vi "pp2_updateSideState.vi"(8 "error in (no error)":errorcluster, 9 "refnum in":refnum<file>, 10 "Daq config In":T1={"Sound AO"="Dev2/ao0", "Shock intesity AO"="Dev1/ao1", "Code_LED DO"="Dev1/port1:2", "Switch DI"="Dev1/port0/line0:1", "Webcam"="cam0", "Sound AO task"="", "Sound card task"=0, "Shock intensity AO task"="", "Code_LED DO task"="", "Switch DI task"="", "AO <=> Sound card"=FALSE, "Sound card"=0, "sample rate"=8000.0, "Variable shock"=FALSE, "Webcam on"=FALSE, "Tone gate PFI"="/Dev1/PFI1", "Waveform memo"={"t0"=timestamp(0 s since 1904-01-01), "dt"=1.0, "Y"=[]}} {"sample rate" min=8000.0; "Sound card task" format="%.0x"}, 11 "State In":T4={"Curr  tr"=0, "Curr (ms)"=0, "Cum (ms)"=0, "Run loop diff"=0, "Tone countdown (ms)"=0, "Countdown (ms)"=0, "Curr State"=enum."0 NULL", "Prev State"=enum."1 Habituation", "Null"=FALSE, "Sw"=FALSE, "Tone\nGate"=FALSE, "Stim"=FALSE, "Current DAQ DO Int"=0, "Current Loaded Trial"={"Trial Type Number"=1, "Trial Type"=enum."GO", "Trial Weight"=100, "Shock (mA)"=0.3, "Duration (ms)"=0.25, "Sound Type"=enum."04 FM Sweep", "Stim P1"=4000.0, "Stim P2"=0.0, "Stim P3"=0.0, "Stim P4"=2000.0}, "Next Trial (for display purposes)"={"Trial Type Number"=1, "Trial Type"=enum."GO", "Trial Weight"=100, "Shock (mA)"=0.3, "Duration (ms)"=0.25, "Sound Type"=enum."04 FM Sweep", "Stim P1"=4000.0, "Stim P2"=0.0, "Stim P3"=0.0, "Stim P4"=2000.0}, "Total trials memo"=0, "State start cum memo (ms)"=0, "Last dur jump time memo (ms)"=0, "Last dur shock time memo (ms)"=0, "Tone repeat memo"=0, "Webcam on"=FALSE, "Webcam recording"=FALSE} {"Current DAQ DO Int" format="%b"; "Next Trial (for display purposes)"."Shock (mA)" min=-1.0 max=5.0; "Next Trial (for display purposes)"."Trial Weight" step=1; "Next Trial (for display purposes)"."Duration (ms)" min=0.0 max=1.0; "Next Trial (for display purposes)"."Trial Type Number" min=1 step=1; "Current Loaded Trial"."Shock (mA)" min=-1.0 max=5.0; "Current Loaded Trial"."Trial Weight" step=1; "Current Loaded Trial"."Duration (ms)" min=0.0 max=1.0; "Current Loaded Trial"."Trial Type Number" min=1 step=1}) -> (0 "error out":errorcluster, 2 "Daq config Out":T1={"Sound AO"="Dev2/ao0", "Shock intesity AO"="Dev1/ao1", "Code_LED DO"="Dev1/port1:2", "Switch DI"="Dev1/port0/line0:1", "Webcam"="cam0", "Sound AO task"="", "Sound card task"=0, "Shock intensity AO task"="", "Code_LED DO task"="", "Switch DI task"="", "AO <=> Sound card"=FALSE, "Sound card"=0, "sample rate"=8000.0, "Variable shock"=FALSE, "Webcam on"=FALSE, "Tone gate PFI"="/Dev1/PFI1", "Waveform memo"={"t0"=timestamp(0 s since 1904-01-01), "dt"=1.0, "Y"=[]}} {"sample rate" min=8000.0; "Sound card task" format="%.0x"}, 3 "State Out":T4={"Curr  tr"=0, "Curr (ms)"=0, "Cum (ms)"=0, "Run loop diff"=0, "Tone countdown (ms)"=0, "Countdown (ms)"=0, "Curr State"=enum."0 NULL", "Prev State"=enum."1 Habituation", "Null"=FALSE, "Sw"=FALSE, "Tone\nGate"=FALSE, "Stim"=FALSE, "Current DAQ DO Int"=0, "Current Loaded Trial"={"Trial Type Number"=1, "Trial Type"=enum."GO", "Trial Weight"=100, "Shock (mA)"=0.3, "Duration (ms)"=0.25, "Sound Type"=enum."04 FM Sweep", "Stim P1"=4000.0, "Stim P2"=0.0, "Stim P3"=0.0, "Stim P4"=2000.0}, "Next Trial (for display purposes)"={"Trial Type Number"=1, "Trial Type"=enum."GO", "Trial Weight"=100, "Shock (mA)"=0.3, "Duration (ms)"=0.25, "Sound Type"=enum."04 FM Sweep", "Stim P1"=4000.0, "Stim P2"=0.0, "Stim P3"=0.0, "Stim P4"=2000.0}, "Total trials memo"=0, "State start cum memo (ms)"=0, "Last dur jump time memo (ms)"=0, "Last dur shock time memo (ms)"=0, "Tone repeat memo"=0, "Webcam on"=FALSE, "Webcam recording"=FALSE} {"Current DAQ DO Int" format="%b"; "Next Trial (for display purposes)"."Shock (mA)" min=-1.0 max=5.0; "Next Trial (for display purposes)"."Trial Weight" step=1; "Next Trial (for display purposes)"."Duration (ms)" min=0.0 max=1.0; "Next Trial (for display purposes)"."Trial Type Number" min=1 step=1; "Current Loaded Trial"."Shock (mA)" min=-1.0 max=5.0; "Current Loaded Trial"."Trial Weight" step=1; "Current Loaded Trial"."Duration (ms)" min=0.0 max=1.0; "Current Loaded Trial"."Trial Type Number" min=1 step=1}, 4 "State timeout":bool, 6 "Side change":bool)   [LabVIEW 2013]
uses:
  pp2_CTL_StateInfo.ctl
  pp2_CTL_State.ctl
  pp2_Trial.ctl
  pp2_CTL_TrialType.ctl
  labolabo2/waveforms/WFTypes.ctl
  pp2_CTL_DaqConfig.ctl
  <vilib>/userdefined/High Color/IMAQdx.ctl
  <vilib>/sound2/lvsound2.llb/Sound Output Task ID.ctl
  <vilib>/DAQmx/read.llb/DAQmx Read (Digital Bool 1Line 1Point).vi
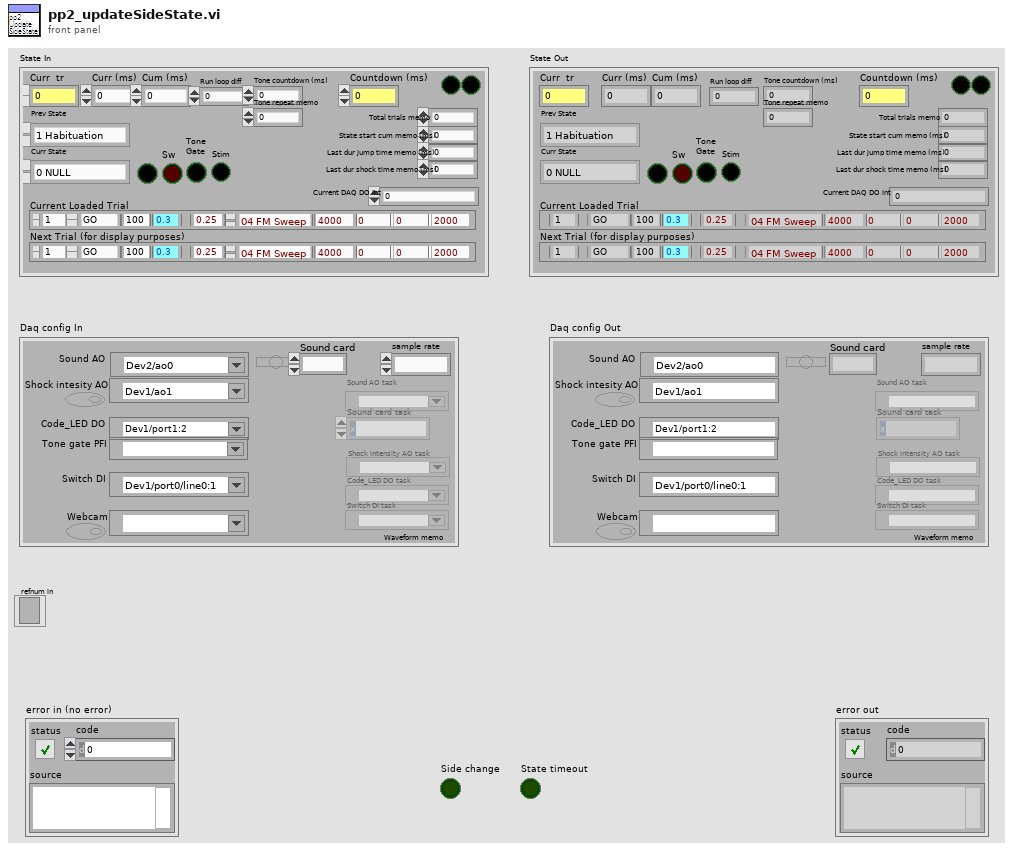
[diagram p1: front panel]
types:
  T1 = typedef "pp2_CTL_DaqConfig.ctl" = cluster{"Sound AO":tag, "Shock intesity AO":tag, "Code_LED DO":tag, "Switch DI":tag, "Webcam":T2, "Sound AO task":refnum<k21>, "Sound card task":T3, "Shock intensity AO task":refnum<k21>, "Code_LED DO task":refnum<k21>, "Switch DI task":refnum<k21>, "AO <=> Sound card":bool, "Sound card":u32, "sample rate":dbl, "Variable shock":bool, "Webcam on":bool, "Tone gate PFI":tag, "Waveform memo":waveform(dbl)}
  T2 = typedef "IMAQdx.ctl" = refnum<k21>
  T3 = typedef "Sound Output Task ID.ctl" = u32
  T4 = typedef "pp2_CTL_StateInfo.ctl" = cluster{"Curr  tr":u16, "Curr (ms)":i64, "Cum (ms)":i64, "Run loop diff":i64, "Tone countdown (ms)":i64, "Countdown (ms)":i64, "Curr State":T5, "Prev State":T5, "Null":bool, "Sw":bool, "Tone\nGate":bool, "Stim":bool, "Current DAQ DO Int":u16, "Current Loaded Trial":T6, "Next Trial (for display purposes)":T6, "Total trials memo":i64, "State start cum memo (ms)":i64, "Last dur jump time memo (ms)":i64, "Last dur shock time memo (ms)":i64, "Tone repeat memo":i64, "Webcam on":bool, "Webcam recording":bool}
  T5 = typedef "pp2_CTL_State.ctl" = enum8{"0 NULL", "1 Habituation", "2 (Load Trial)", "3 Stay Period", "4 Load Audio/Click Delay", "5 GO Trial", "6 GO Jumped", "7 GO Timeout", "8 NOGO Trial", "9 NOGO Jumped", "10 NOGO Timeout", "11 TEST Trial", "12 TEST Jumped", "13 TEST Timeout", "14 Intertrial Interval", "15 Done"}
  T6 = typedef "pp2_Trial.ctl" = cluster{"Trial Type Number":u8, "Trial Type":T7, "Trial Weight":u32, "Shock (mA)":dbl, "Duration (ms)":dbl, "Sound Type":T8, "Stim P1":dbl, "Stim P2":dbl, "Stim P3":dbl, "Stim P4":dbl}
  T7 = typedef "pp2_CTL_TrialType.ctl" = enum16{"OFF", "GO", "NOGO", "TEST"}
  T8 = typedef "WFTypes.ctl" = enum16{"00 NULL", "01 DC", "02 Noise", "03 Pure Tone", "04 FM Sweep"}
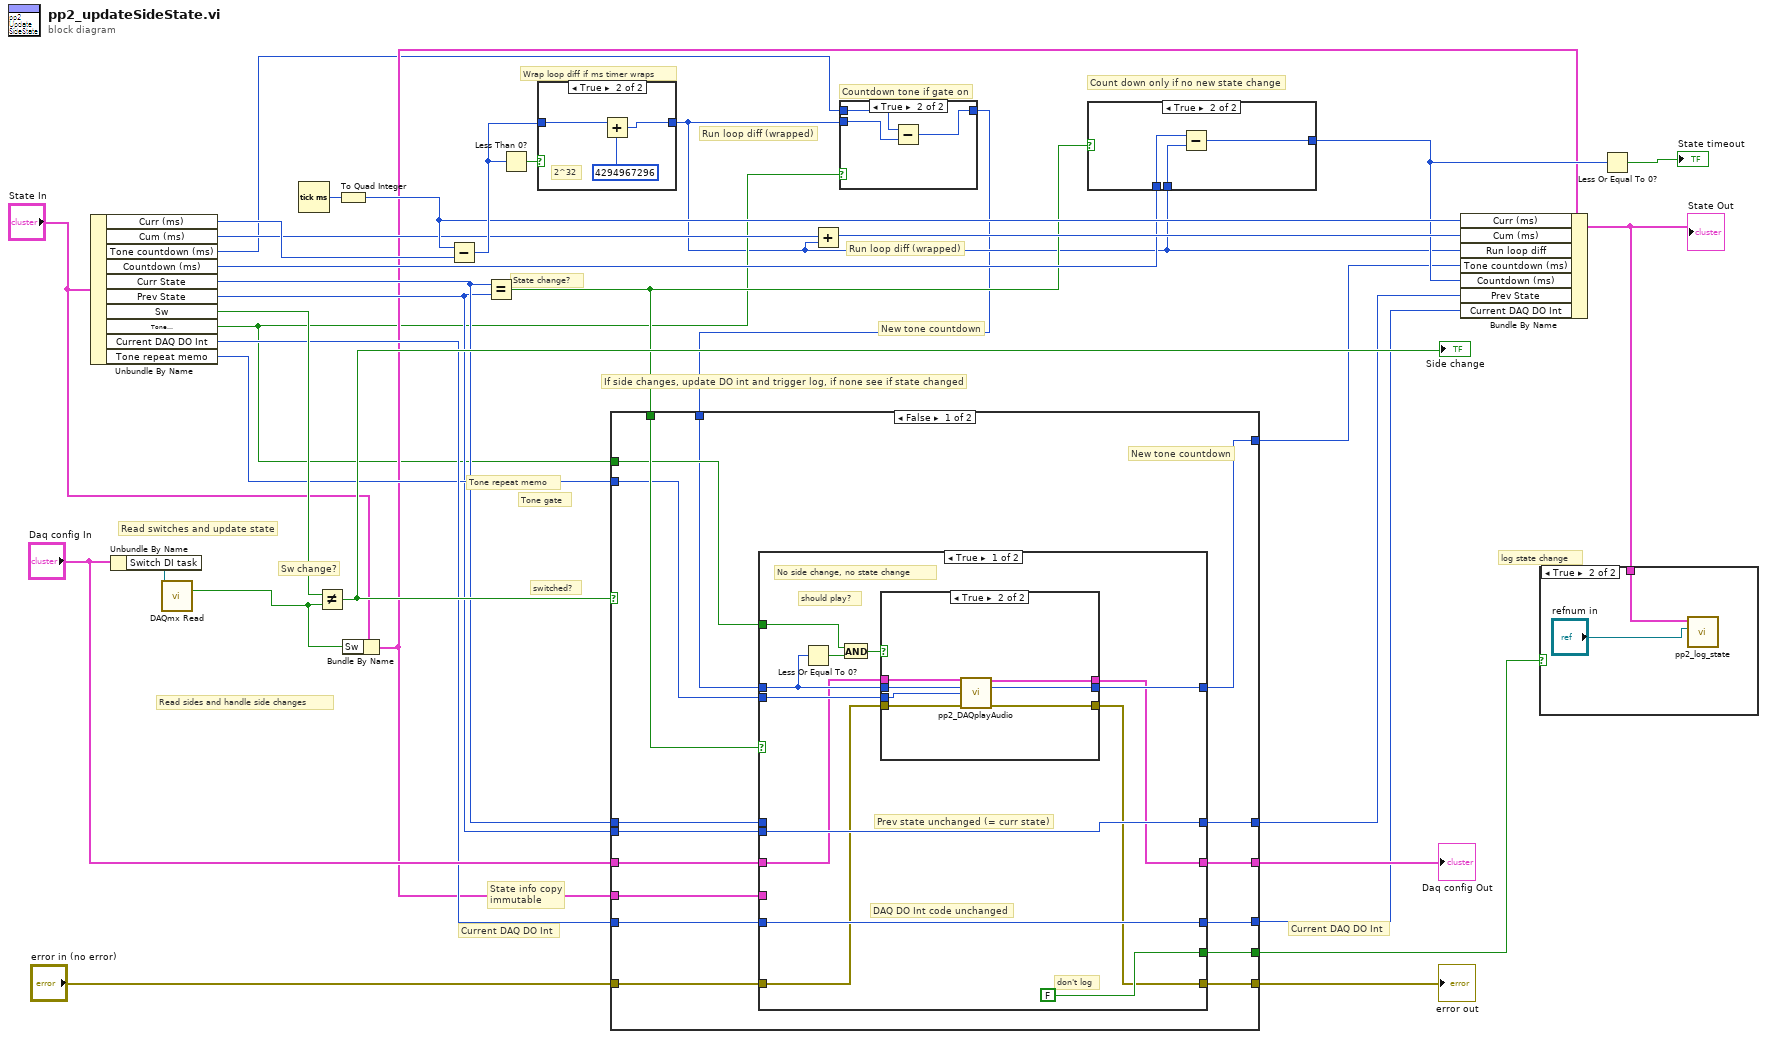
[diagram p0: block diagram]
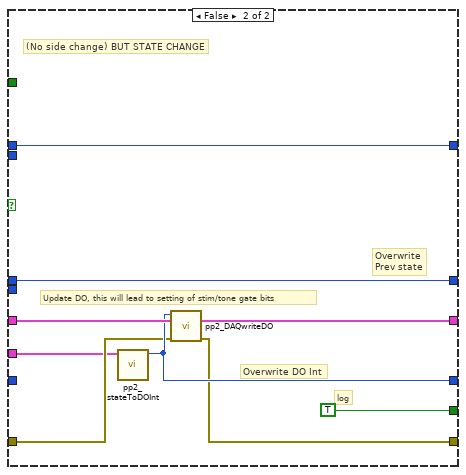
[diagram p6: hidden frame]
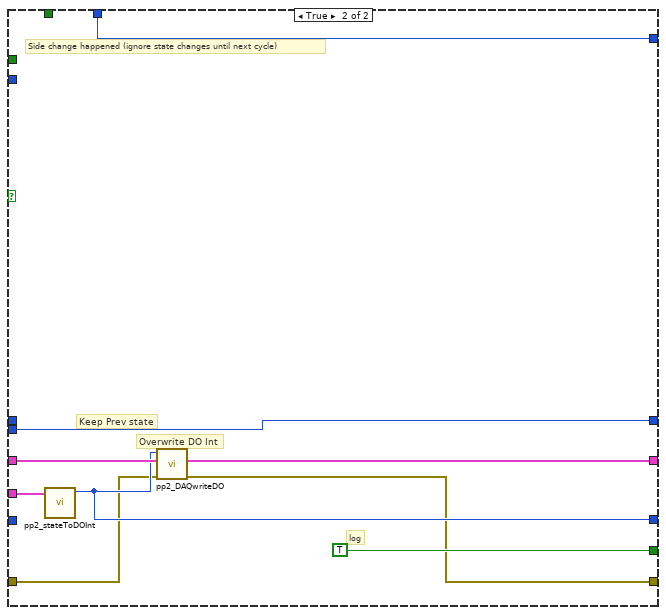
[diagram p7: hidden frame]
diagram:
  # "New tone countdown"
  # "Countdown tone if gate on"
  # "switched?"
  # "Read switches and update state"
  # "State info copy\nimmutable"
  # "Tone repeat memo"
  # "Sw change?"
  # "Run loop diff (wrapped)"
  # "State change?"
  # "Current DAQ DO Int"
  # "Current DAQ DO Int"
  # "Count down only if no new state change"
  # "Tone gate"
  # "Run loop diff (wrapped)"
  # "Wrap loop diff if ms timer wraps"
  # "If side changes, update DO int and trigger log, if none see if state changed"
  # "Read sides and handle side changes"
  # "log state change"
  n1 = Unbundle By Name("State In") -> ("Curr (ms)"=w30:i64, "Cum (ms)"=w29:i64, "Tone countdown (ms)"=w3:i64, "Countdown (ms)"=w27:i64, "Curr State"=w12:T5, "Prev State"=w11:T5, "Sw"=w25:bool, "Tone\nGate"=w5:bool, "Current DAQ DO Int"=w18:u16, "Tone repeat memo"=w13:i64)
  n2 = Unbundle By Name("Daq config In") -> ("Switch DI task"=w26:refnum<k21>)
  n3 = call-poly <vilib>:"DAQmx Read.vi"("task/channels in"=w26) -> ("data"=w1:bool)  [unwired: 12 in, 2 out]
  n4 = Tick Count (ms)() -> (millisecond timer value=w34:u32)
  n5 = Not Equal?(x=w25, y=w1) -> (x != y?=w22:bool)
  "Side change" <- w22
  n6 = To Quad Integer(1:w34) -> (0:w31:i64)
  n7 = Bundle By Name(cluster="State In", "Sw"=w1) -> (w6:T4)
  n8 = Subtract(x=w31, y=w30) -> (x-y=w32:i64)
  n9 = Equal?(x=w12, y=w11) -> (x = y?=w10:bool)
  n10 = Less Than 0?(x=w32) -> (x < 0?=w33:bool)
  n11 = case shown="True" w33 {
    tunnel: w32 -> [w35 w37]
    tunnel: [w35 w38] -> w4
    frame False {
    }
    frame True {
      # "2^32"
      n12 = Add(x=w37, y=i64 4294967296) -> (x+y=w38:i64)
    }
  }
  n13 = Add(x=w29, y=w4) -> (x+y=w28:i64)
  n14 = case shown="True" w5 {
    tunnel: [w39 w40] -> w2
    tunnel: w3 -> [w39 w42]
    tunnel: w4 -> [_ w41]
    frame False {
      # "Passthrough if\ntone gate off"
    }
    frame True {
      n15 = Subtract(x=w42, y=w41) -> (x-y=w40:i64)
    }
  }
  n16 = case shown="False" w22 {
    tunnel: w12 -> [w58 _]
    tunnel: w11 -> [w56 w99]
    tunnel: [w57 w99] -> w21
    tunnel: "Daq config In" -> [w48 w97]
    tunnel: [w54 w95] -> w7
    tunnel: [w53 w96] -> w19
    tunnel: w18 -> [w55 _]
    tunnel: "error in (no error)" -> [w47 w94]
    tunnel: [w51 w93] -> w16
    tunnel: [w52 TRUE] -> w15
    tunnel: w5 -> [w44 _]
    tunnel: w13 -> [w46 _]
    tunnel: w10 -> [w50 _]
    tunnel: w6 -> [w49 w92]
    tunnel: [w45 w91] -> w9
    tunnel: w2 -> [w43 w91]
    frame False {
      # "New tone countdown"
      n17 = case shown="True" w50 {
        tunnel: w58 -> [_ w90]
        tunnel: [w71 w90] -> w57
        tunnel: w56 -> [w71 _]
        tunnel: w55 -> [w70 _]
        tunnel: [w70 w87] -> w54
        tunnel: w48 -> [w65 w89]
        tunnel: [w64 w88] -> w53
        tunnel: [FALSE TRUE] -> w52
        tunnel: w47 -> [w62 w85]
        tunnel: [w63 w84] -> w51
        tunnel: w49 -> [_ w83]
        tunnel: w43 -> [w67 w82]
        tunnel: w46 -> [w68 _]
        tunnel: [w66 w82] -> w45
        tunnel: w44 -> [w59 _]
        frame True {
          # "should play?"
          # "don't log"
          # "DAQ DO Int code unchanged"
          # "No side change, no state change"
          # "Prev state unchanged (= curr state)"
          n18 = Less Or Equal To 0?(x=w67) -> (x <= 0?=w60:bool)
          n19 = And(x=w59, y=w60) -> (x .and. y?=w61:bool)
          n20 = case shown="True" w61 {
            tunnel: [w74 w81] -> w64
            tunnel: [w73 w80] -> w63
            tunnel: w67 -> [w72 w79]
            tunnel: w68 -> [_ w78]
            tunnel: [w72 w77] -> w66
            tunnel: w65 -> [w74 w76]
            tunnel: w62 -> [w73 w75]
            frame False {
            }
            frame True {
              n21 = call "pp2_DAQplayAudio.vi"("Daq config In"=w76, "Tone countdown (ms) In"=w79, "Tone repeat memo"=w78, "error in (no error)"=w75) -> ("Daq config Out"=w81:T1, "Tone countdown (ms) Out"=w77:i64, "error out"=w80:errorcluster)  [unwired: 9 in]
            }
          }
        }
        frame False {
          # "log"
          # "Overwrite DO Int"
          # "Update DO, this will lead to setting of stim/tone gate bits"
          # "(No side change) BUT STATE CHANGE"
          # "Overwrite\nPrev state"
          n22 = call "pp2_stateToDOInt.vi"("State In"=w83) -> ("DAQ Output Int"=w87:u16)  [unwired: 10 in]
          n23 = call "pp2_DAQwriteDO.vi"("error in (no error)"=w85, "Daq config"=w89, "DAQ Digital In"=w87) -> ("error out"=w84:errorcluster, "Daq config 2"=w88:T1)  [unwired: 7 in]
        }
      }
    }
    frame True {
      # "log"
      # "Side change happened (ignore state changes until next cycle)"
      # "Overwrite DO Int"
      # "Keep Prev state"
      n24 = call "pp2_stateToDOInt.vi"("State In"=w92) -> ("DAQ Output Int"=w95:u16)  [unwired: 10 in]
      n25 = call "pp2_DAQwriteDO.vi"("error in (no error)"=w94, "Daq config"=w97, "DAQ Digital In"=w95) -> ("error out"=w93:errorcluster, "Daq config 2"=w96:T1)  [unwired: 7 in]
    }
  }
  "Daq config Out" <- w19
  "error out" <- w16
  n26 = case shown="True" w10 {
    tunnel: w27 -> [w100 w103]
    tunnel: [w100 w102] -> w24
    tunnel: w4 -> [_ w101]
    frame False {
      # "Passthrough if new state change"
    }
    frame True {
      n27 = Subtract(x=w103, y=w101) -> (x-y=w102:i64)
    }
  }
  n28 = Bundle By Name(cluster=w6, "Curr (ms)"=w31, "Cum (ms)"=w28, "Run loop diff"=w4, "Tone countdown (ms)"=w9, "Countdown (ms)"=w24, "Prev State"=w21, "Current DAQ DO Int"=w7) -> (w14:T4)
  "State Out" <- w14
  n29 = case shown="True" w15 {
    tunnel: w14 -> [_ w105]
    frame False {
    }
    frame True {
      n30 = call "pp2_log_state.vi"("refnum in"="refnum in", "State In"=w105) -> ()  [unwired: 10 in]
    }
  }
  n31 = Less Or Equal To 0?(x=w24) -> (x <= 0?=→"State timeout":bool)
